vi "CarWashTest.vi"(0 "VI Reference In":refnum<vi>, 2 "Label":string, 5 "Wash Option":string, 7 "Car Position":i32=1, 9 "Elapsed Time":dbl=5.0, 11 "error in":errorcluster) -> (4 "VI Reference Out":refnum<vi>, 15 "error out":errorcluster)   [LabVIEW 2016, in "CarWashTest.lvlib"]
doc: "Wash test"
uses:
  CarWashTest.lvlib
  APIs/Stimulus/VI/OpenVIFrontPanel.vi
  APIs/Stimulus/ControlValue/ValueSignalByPathString.vi
  APIs/Stimulus/ControlValue/ValueSignalLatchBooleanString.vi
  APIs/Assert/AssertControlDisable/AssertDisabledAndGrayedOut.vi
  APIs/Assert/AssertControlValue/True.vi
  APIs/Stimulus/ControlValue/SetValueAuto.vi
  APIs/Assert/AssertControlValue/Equal.vi
  APIs/Assert/AssertControlValue/AlmostEqual.vi
  <vilib>/addons/_JKI Toolkits/Caraya/classes/Assert/Assert Almost Equal_Float.vi
  Drona.lvlib
  <vilib>/addons/_JKI Toolkits/Caraya/classes/Test/Test.lvclass
  APIs/Assert/AssertControlValue/AssertControlValue.lvlib
  <vilib>/addons/_JKI Toolkits/Caraya/classes/Assert/Assert.lvclass
  APIs/Assert/AssertControlDisable/AssertControlDisable.lvlib
  APIs/Stimulus/ControlValue/ControlValue.lvlib
  APIs/Stimulus/VI/VI.lvlib
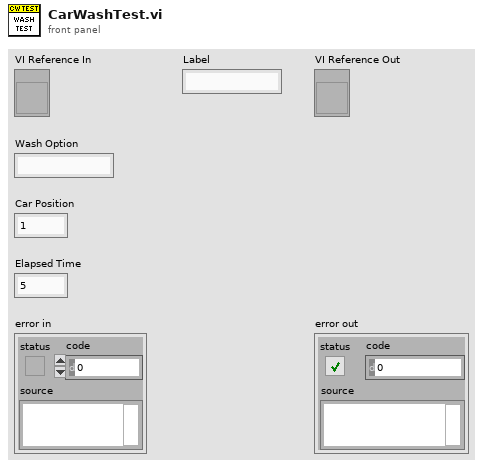
[diagram p1: front panel]
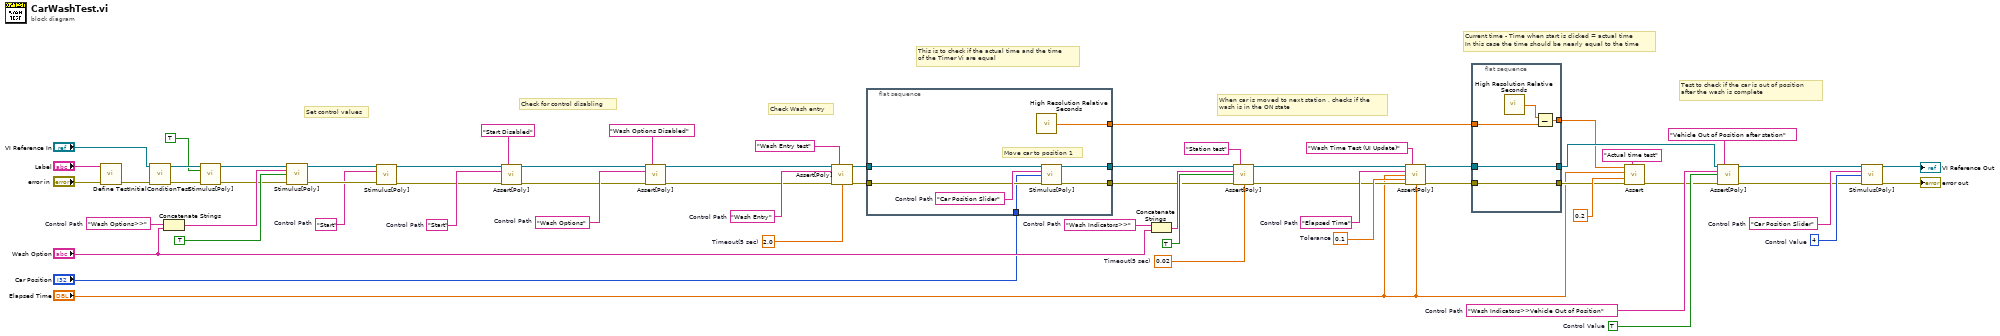
[diagram p0: block diagram]
diagram:
  w9 = "Start"  # Control Path
  w10 = "Wash Options"  # Control Path
  w36 = "Wash Indicators>>"  # Control Path
  w37 = "Start"  # Control Path
  w41 = "Wash Options>>"  # Control Path
  w47 = 4  # Control Value
  w48 = "Car Position Slider"  # Control Path
  w51 = TRUE  # Control Value
  w58 = 0.02  # Timeout(5 sec)
  w55 = 0.1  # Tolerance
  w56 = "Elapsed Time"  # Control Path
  w52 = "Wash Indicators>>Vehicle Out of Position"  # Control Path
  w62 = 2.0  # Timeout(5 sec)
  w63 = "Wash Entry"  # Control Path
  # "Check Wash entry"
  # "Check for control disabling"
  # "Current time - Time when start is clicked = actual time\nIn this case the time should be nearly equal to the time"
  # "This is to check if the actual time and the time \nof the Timer Vi are equal"
  # "Set control values"
  # "Test to check if the car is out of position \nafter the wash is complete"
  # "When car is moved to next station , checks if the\nwash is in the ON state"
  n1 = call <vilib>:"Define Test.vi"("error in (no error)"="error in", "Label (VI Title)"="Label") -> ("error out"=w27:errorcluster)  [unwired: 9 in]
  n2 = call "InitialConditionTest.vi"("VI Reference In"="VI Reference In", "error in"=w27) -> ("VI Reference Out"=w15:refnum<vi>, "error out"=w13:errorcluster)  [unwired: 12 in]
  n3 = Concatenate Strings(w41, "Wash Option") -> (w43:string)
  n4 = call-poly "Stimulus[Poly].vi"("VI Reference In"=w15, "Activate (F)"=TRUE ("Wait Until Done (F)"), "error in"=w13) -> ("VI Reference Out"=w14:refnum<vi>, "error out"=w12:errorcluster)  [unwired: 11 in]
  n5 = call-poly "Stimulus[Poly].vi"("VI Reference In"=w14, "Control Path"=w43, "Value (Signaling)"=TRUE, "error in"=w12) -> ("VI Reference Out"=w39:refnum<vi>, "error out"=w40:errorcluster)  [unwired: 10 in]
  n6 = call-poly "Stimulus[Poly].vi"("VI Reference In"=w39, "Control Path"=w37, "error in"=w40) -> ("VI Reference Out"=w5:refnum<vi>, "error out"=w2:errorcluster)  [unwired: 11 in]
  n7 = call-poly "Assert[Poly].vi"("VI Reference In"=w5, "Test Label"="Start Disabled", "Control Path"=w9, "Error In"=w2) -> ("VI Reference Out"=w7:refnum<vi>, "Error Out"=w8:errorcluster)  [unwired: 9 in, 1 out]
  n8 = call-poly "Assert[Poly].vi"("VI Reference In"=w7, "Test Label"="Wash Options Disabled", "Control Path"=w10, "Error In"=w8) -> ("VI Reference Out"=w4:refnum<vi>, "Error Out"=w3:errorcluster)  [unwired: 9 in, 1 out]
  n9 = call-poly "Assert[Poly].vi"("VI Reference In"=w4, "Test Label"="Wash Entry test" ("Label"), "Control Path"=w63, "Error In"=w3, "Timeout(5 sec)"=w62) -> ("VI Reference Out"=w60:refnum<vi>, "Error Out"=w61:errorcluster)  [unwired: 8 in, 1 out]
  n10 = flat-sequence {
    tunnel: w61 -> [w69]
    tunnel: w60 -> [w68]
    tunnel: [w67] -> w49
    tunnel: "Car Position" -> [w66]
    tunnel: [w65] -> w30
    tunnel: [w64] -> w22
    frame #0 {
      w70 = "Car Position Slider"  # Control Path
      # "Move car to position 1"
      n11 = call <vilib>:"High Resolution Relative Seconds.vi"() -> ("relative seconds"=w64:dbl)
      n12 = call-poly "Stimulus[Poly].vi"("VI Reference In"=w68, "Control Path"=w70, "Value (Signaling)"=w66, "error in"=w69) -> ("VI Reference Out"=w67:refnum<vi>, "error out"=w65:errorcluster)  [unwired: 10 in]
    }
  }
  n13 = Concatenate Strings(w36, "Wash Option") -> (w35:string)
  n14 = call-poly "Assert[Poly].vi"("VI Reference In"=w49, "Test Label"="Station test" ("Label"), "Control Path"=w35, "Control Value"=TRUE, "Error In"=w30, "Timeout(5 sec)"=w58) -> ("VI Reference Out"=w54:refnum<vi>, "Error Out"=w31:errorcluster)  [unwired: 7 in, 1 out]
  n15 = call-poly "Assert[Poly].vi"("VI Reference In"=w54, "Test Label"="Wash Time Test (UI Update)" ("Label"), "Control Path"=w56, "Control Value"="Elapsed Time", "Tolerance"=w55, "Error In"=w31, "Timeout(5 sec)"="Elapsed Time") -> ("VI Reference Out"=w24:refnum<vi>, "Error Out"=w25:errorcluster)  [unwired: 6 in, 1 out]
  n16 = flat-sequence {
    tunnel: [w75] -> w17
    tunnel: w25 -> [w75]
    tunnel: [w74] -> w23
    tunnel: w24 -> [w74]
    tunnel: w22 -> [w72]
    tunnel: [w71] -> w19
    frame #0 {
      n17 = call <vilib>:"High Resolution Relative Seconds.vi"() -> ("relative seconds"=w73:dbl)
      n18 = Subtract(x=w73, y=w72) -> (x-y=w71:dbl)
    }
  }
  n19 = call-poly <vilib>:"Assert.vi"("Label"="Actual time test", "error in (no error)"=w17, "Tolerance"=0.2, "Y"="Elapsed Time", "X"=w19) -> ("error out"=w18:errorcluster)  [unwired: 6 in]
  n20 = call-poly "Assert[Poly].vi"("VI Reference In"=w23, "Test Label"="Vehicle Out of Position after station" ("Label"), "Control Path"=w52, "Control Value"=w51, "Error In"=w18) -> ("VI Reference Out"=w46:refnum<vi>, "Error Out"=w45:errorcluster)  [unwired: 8 in, 1 out]
  n21 = call-poly "Stimulus[Poly].vi"("VI Reference In"=w46, "Control Path"=w48, "Value (Signaling)"=w47, "error in"=w45) -> ("VI Reference Out"=→"VI Reference Out":refnum<vi>, "error out"=→"error out":errorcluster)  [unwired: 10 in]
